vi "Main_02a.vi"() -> ()   [LabVIEW 2020]
uses:
  ENUM RPS Select.ctl
panel:
  in  "Example":string="A Y\nC Y\nC X\nA Y\nC X\nC Y\nB Z\nA Y\nA Y\nC Z\nA Y\nA Y\nA Y\nC Y\nA Y\nA Y\nA Y\nA X\nB X\nA X\nA Y\nC Y\nC X\nA Y\nA Y\nC Y\nA X\nA Y\nB Z\nA Y\nC X\nA Y\nA Y\nC Z\nC Y\nC X\nA Y\nA Z\nA Y\nA Y\nA Y\nA Y\nC Y\nC Y\nB Z\nB Z\nC Y\nB X\nA Y\nA Y\nA Y\nC Z\nA Y\nC X\nA Z\nC Y\nA Y\nA Y\nA Y\nA Y\nA Y\nC X\nA Y\nC Y\nA Y\nC Y\nA Y\nA X\nC Y\nA X\nA Y\nC Y\nC Y\nA Y\nC X\nA Y\nA Y\nA Y\nC X\nA Y\nA Y\nA Y\nC X\nA Y\nC X\nA Y\nA Y\nC Z\nA Y\nA Y\nA Y\nC X\nA Y\nA X\nC Y\nA X\nB Z\nC Y\nA Y\nA Y\nB Z\nC Y\nA Y\nA Z\nC Z\nC Y\nB Z\nA Y\nA Y\nC Y\nA Y\nC X\nA Y\nA Y\nC X\nC X\nC Y\nA Y\nA Y\nC X\nA Y\nA Y\nA Y\nA Y\nC X\nC Y\nA Y\nA Y\nA Y\nC Z\nA Y\nC Y\nA Y\nC X\nC Z\nA Y\nB X\nA Y\nC X\nA Y\nB X\nA Y\nC Z\nA Y\nA Y\nA Y\nA X\nA Y\nA Y\nA Y\nC Y\nA Y\nA Y\nA Y\nA Y\nC Y\nC X\nA Y\nA Y\nA Y\nA Y\nC Y\nA Y\nA Y\nA Y\nC Y\nB X\nA Y\nA Y\nA Y\nA Y\nA Y\nA X\nC Y\nA Y\nC X\nA X\nB Y\nA Y\nC X\nA Y\nC Y\nC Y\nA Z\nC Z\nC X\nB X\nC Y\nA Y\nC Z\nA Z\nA Y\nC X\nA Y\nA Y\nC X\nA Y\nB X\nC X\nA Z\nC Y\nA Y\nC X\nA Y\nA Y\nA Y\nB Z\nC Z\nA Y\nA X\nC X\nA Y\nA Y\nC Y\nA Y\nA Y\nA X\nA X\nC Y\nC X\nB X\nA Y\nA Y\nA Y\nA Y\nB Y\nA Y\nC Y\nA Y\nA X\nB Z\nA X\nC Z\nC X\nC X\nC Y\nC X\nC X\nA X\nC X\nA Y\nC Y\nA X\nC X\nB Z\nC Z\nA Y\nC X\nB Y\nA Z\nC Y\nC X\nA Y\nA Y\nA Y\nC X\nA Y\nA Y\nA Y\nA X\nB Y\nC Y\nC X\nB Z\nA Y\nA Y\nB Y\nA Y\nA Y\nA Y\nC X\nA Y\nA Y\nA Y\nA Y\nA Y\nA Y\nA Y\nA Y\nA Y\nC Y\nC Y\nC Z\nA Y\nC Y\nA Y\nA Y\nA X\nA X\nA Y\nA Y\nC Y\nA Y\nA X\nA Y\nA Y\nC X\nA Y\nC X\nC X\nC Y\nB Y\nA Y\nC X\nA Y\nA Y\nA X\nA Y\nA Y\nA X\nA Y\nB Z\nC Y\nA Y\nA Y\nA Y\nC Y\nC Z\nA Y\nA Y\nA Y\nA Y\nA Y\nC Y\nC Y\nC Y\nC Y\nC Y\nA X\nC Y\nA Y\nA Y\nA Y\nA Y\nC X\nA Y\nC Z\nA Y\nB Y\nA X\nA Y\nA Y\nA Y\nC Y\nC Y\nA X\nC Y\nA Y\nA Y\nA Y\nB Z\nA X\nA Y\nA Y\nA Z\nC Y\nA Y\nC X\nC Y\nC Y\nC Z\nB Y\nC X\nC X\nA Z\nC Y\nA Y\nA Z\nA X\nA Z\nC Y\nC X\nB Z\nA X\nC Y\nA Y\nC Y\nB Z\nA Y\nA Y\nC X\nC X\nC X\nA Y\nB X\nC X\nC Y\nC X\nA X\nA X\nB X\nA Y\nA Y\nA Y\nC X\nA Y\nC Y\nC X\nA Y\nB Z\nA Y\nA Y\nA Y\nB X\nA Y\nA Y\nA Y\nC Y\nA Y\nC X\nC Y\nC Y\nA Y\nB Z\nC Y\nC X\nC Y\nC X\nC X\nC Y\nA Y\nA Z\nA Y\nA Y\nA Y\nA Y\nC Z\nA Y\nA Y\nC Y\nA Y\nA X\nC Z\nC Y\nC X\nC X\nA Y\nA Z\nA Z\nB Y\nA X\nC X\nC X\nA Y\nA Y\nA Y\nC Z\nC X\nC X\nC X\nA Y\nC Z\nA Z\nC X\nC Y\nA X\nC X\nC X\nA Y\nC Y\nC Y\nB X\nB Z\nA Y\nA Y\nA Y\nB Z\nC Y\nA Y\nB Z\nA X\nC Y\nC Y\nB X\nC X\nB Y\nA Y\nB X\nC Z\nA Y\nA Z\nC Z\nC Z\nA Y\nA X\nA Y\nA X\nC Y\nA Y\nA Y\nA Y\nC X\nC X\nC X\nA Y\nA Y\nA Y\nA Y\nA Y\nC Y\nA Y\nC Y\nA Z\nC X\nC Y\nA Y\nA Y\nB Y\nC Y\nA Y\nC Z\nC Z\nA Y\nB Y\nA Y\nA Y\nA X\nC Y\nA Y\nA Y\nA Y\nC Z\nC Y\nC X\nA Y\nA Y\nB Z\nC Y\nC X\nC Z\nA Y\nC Y\nA Y\nA Y\nC X\nC Y\nC Y\nA Y\nC Y\nC X\nC Y\nA Y\nA Y\nA Y\nA Z\nB Z\nA Y\nA Y\nA X\nC Z\nC X\nA Y\nA Y\nA Y\nC X\nC Y\nB Z\nC X\nA Y\nA Y\nA Y\nC Y\nA Y\nC X\nC Z\nC X\nA Y\nA X\nA Y\nC Z\nC X\nB Y\nA Y\nA X\nA Y\nB Y\nA Y\nA Y\nC Y\nC Z\nC Y\nC Y\nC X\nA Y\nA Y\nA X\nA Y\nA Y\nA Z\nA X\nC Y\nA Y\nC Y\nC Y\nC Z\nC Y\nC Y\nA Z\nA Y\nC Z\nC Y\nC Y\nC Y\nB X\nC Y\nA Y\nC X\nA Y\nB X\nC Z\nC Z\nC Y\nA Y\nC X\nA Y\nA Y\nA Y\nA Y\nC Z\nA Z\nA X\nC Y\nC X\nA Y\nA Y\nC X\nC Y\nC Z\nC X\nC Y\nA X\nA Y\nA Y\nB X\nA Y\nA X\nC X\nA Y\nA Y\nA Y\nB Z\nA Z\nB Z\nC X\nB Z\nA Y\nC X\nA Y\nC X\nA Y\nA Y\nC Y\nA Y\nA Y\nB X\nA Y\nC Y\nA Y\nA Y\nA Y\nC Y\nA Y\nA Y\nA Y\nB Y\nA Y\nC Y\nA Y\nA Y\nA Y\nA Y\nC Y\nA X\nB X\nA Y\nB Z\nC X\nA X\nB X\nC Y\nA Y\nB X\nC Y\nA Y\nB X\nA Y\nC X\nB X\nA Y\nA Y\nA Y\nA Y\nC X\nC X\nA Y\nB X\nC Y\nA Y\nA Y\nA Y\nA Y\nB X\nA Y\nB Z\nC X\nA Y\nB Z\nC X\nC Z\nC Z\nB X\nC Y\nA Y\nA Y\nA Y\nA Y\nA Y\nA Y\nC Y\nA Y\nA Y\nA X\nA X\nC X\nA Y\nC Z\nC Y\nA Y\nC X\nA Z\nA Z\nA Y\nC Z\nA Y\nA Y\nA Y\nC Y\nA X\nC X\nC Z\nA Y\nA Y\nC X\nB X\nA Y\nA Z\nC Y\nA Z\nA Y\nA Y\nA Y\nA Y\nA Y\nB X\nA Y\nC Y\nC X\nA Y\nA Y\nC Z\nC Z\nC Y\nA Y\nB Z\nA Y\nA Y\nA Y\nA Y\nA Y\nC X\nA Z\nA Y\nC Y\nA Z\nC X\nA Y\nC X\nA Y\nA Y\nC Z\nC Y\nA Y\nA Z\nC X\nC X\nA Y\nB Z\nA Y\nB X\nC Y\nC X\nC Z\nA Y\nA X\nC X\nC Z\nC Y\nC X\nA Y\nA Y\nA Y\nA Y\nA Y\nA Y\nC Y\nA Y\nC Y\nA Y\nC Y\nB Y\nA Y\nA Y\nA Y\nA Y\nB Z\nC Y\nA Y\nC Y\nA X\nC Y\nA Y\nB Y\nC Y\nC X\nC X\nA Y\nA Y\nA Y\nC X\nA X\nA Y\nA X\nC Y\nA Y\nA Y\nC Y\nC Y\nA Z\nA Y\nA Y\nB X\nA Z\nB X\nA Y\nC Y\nA X\nC Y\nC Z\nB Z\nA Y\nA Y\nC Y\nA Y\nC Z\nA Y\nA X\nA Y\nC Y\nA Y\nA Y\nA Y\nA Y\nA Y\nA Y\nA Y\nA Y\nC X\nC Y\nA Y\nA Z\nA Y\nC X\nA Y\nC Z\nA Y\nC X\nA X\nA Y\nC Y\nA Y\nC X\nA X\nA Y\nA Y\nA Y\nC Y\nA Y\nC Y\nA Y\nB Y\nC Y\nC Y\nA Y\nA Y\nA Y\nA Y\nC Z\nA Y\nC Z\nA Y\nC Y\nB X\nA X\nC Y\nC Z\nA X\nA Z\nA Y\nA X\nC Z\nC Y\nA Z\nC Y\nA X\nA Y\nA Y\nA X\nC Z\nA X\nA Z\nC Y\nA Y\nC Y\nA Z\nB Z\nA Y\nC X\nC X\nA Y\nA Y\nA X\nA Y\nA Y\nA Y\nC X\nA Y\nB X\nA Y\nC X\nA Y\nC Y\nA Y\nC Y\nC Z\nC Y\nC Z\nA Z\nA Y\nC Y\nC Z\nC Z\nA Y\nA Y\nC Y\nA X\nA Y\nC Y\nA Y\nA Y\nA Y\nA X\nA Y\nB Z\nC Y\nC X\nA Y\nC X\nB X\nC Y\nC Y\nA Y\nC Y\nC Y\nA X\nA Y\nA X\nA Y\nA Z\nC Z\nB X\nA Y\nC X\nA Y\nC Z\nA Y\nC Y\nA Z\nA Y\nA Y\nA Y\nC Y\nC Y\nA Y\nA Y\nC Y\nA Y\nC Y\nC Y\nA X\nA Y\nC X\nC Z\nA Y\nA Y\nA Y\nC X\nC X\nC Y\nC Y\nC Z\nA X\nA Y\nC Y\nC Z\nA Y\nB Y\nA Y\nC Z\nC Z\nA Y\nA Y\nA Y\nB Z\nA Y\nA Z\nA X\nC X\nC X\nC Z\nA Y\nC Z\nA Z\nC Y\nC Z\nC X\nC Y\nC X\nA Y\nC Y\nA Z\nA Y\nA Y\nA Y\nA Y\nC Y\nA X\nC X\nA Y\nA Y\nC Z\nB Z\nA Y\nA Y\nC X\nA Y\nC Y\nC Y\nB Z\nA Y\nC Y\nA Y\nC X\nC X\nA Y\nC Y\nA X\nC X\nA Y\nC Z\nA Y\nC X\nA Y\nC X\nA Y\nC Y\nA Y\nC Z\nA Y\nC Z\nA Y\nA Y\nA Y\nC Y\nA Y\nA X\nA Z\nA Y\nC Y\nC Y\nA Y\nA Y\nB Z\nA X\nA X\nC X\nC X\nC Z\nC Z\nA Y\nA Y\nA Y\nA X\nA X\nA Y\nA Z\nC Y\nC Y\nC X\nA Y\nC X\nB X\nA X\nA Z\nA Y\nB X\nA Y\nB Z\nB Z\nA Y\nB X\nC Y\nA Y\nA Y\nC Y\nC Y\nA Y\nA Y\nA Z\nA Y\nC Z\nB X\nA Y\nC Y\nC Y\nA Y\nB X\nC X\nC Y\nA X\nC X\nA Y\nA X\nA Y\nA Y\nB Z\nA X\nC Y\nA Y\nA Z\nB Y\nA Y\nB X\nA Z\nC Y\nC Z\nC Z\nC Z\nC Y\nA Y\nC Y\nC Y\nB Y\nA Y\nC Z\nB Y\nA Y\nA Y\nA Y\nA X\nB Z\nA Y\nC Z\nA Y\nA X\nC Z\nC X\nA Y\nA Y\nA Y\nB Z\nB Z\nA Y\nC Z\nA Y\nA Y\nA Y\nC Y\nC Z\nC X\nA Y\nB Z\nC Y\nB Z\nC X\nC X\nA Y\nA X\nA X\nB Z\nC Y\nC Y\nC X\nA Y\nC X\nC X\nA Y\nC X\nC Z\nA X\nC Y\nC Y\nC Y\nA Y\nA X\nC Y\nA Y\nA Y\nC Y\nC X\nC Y\nB X\nC X\nA Z\nA X\nA Y\nC Y\nA Y\nA X\nC Y\nA Y\nA X\nC X\nA X\nC X\nC Y\nC Y\nA Y\nC X\nA Y\nA X\nC Y\nA Y\nC Z\nA Z\nA Y\nA Y\nA Y\nA Z\nA Y\nB X\nB Z\nC X\nA Z\nC X\nA Y\nA Z\nA X\nC Y\nC Y\nB Z\nA Z\nA Y\nA Y\nA Y\nB X\nC Y\nA Y\nA X\nA Y\nB Z\nB Z\nA Y\nA Y\nA Y\nC X\nC X\nC X\nC Y\nA Y\nC Y\nC Y\nA Y\nA Y\nA Y\nA Y\nC Y\nA Y\nC X\nA Y\nC X\nC Y\nC Y\nC Z\nB X\nA Y\nC Y\nA Y\nC Y\nA Y\nA Y\nA Y\nA Y\nB Z\nC Z\nC Y\nA X\nC Y\nA Y\nC Y\nC Y\nA Y\nB Z\nC Y\nB X\nB X\nA Y\nA Y\nC Y\nC Y\nB X\nA X\nC Y\nC X\nC Y\nA Y\nA Y\nC X\nA X\nA Z\nA Y\nA Z\nA Y\nB X\nA X\nC X\nA X\nC X\nC Z\nA Y\nC X\nC Y\nC X\nC Y\nA Y\nC Y\nA Y\nA Y\nC Y\nC Z\nC X\nA Y\nA Y\nA X\nC Y\nB Z\nA Y\nC Y\nB Z\nC Y\nA Y\nC Y\nA X\nA X\nA Y\nB X\nA Y\nC X\nC Y\nA Y\nA Y\nA Y\nC X\nC Z\nA Y\nC Y\nA Z\nC Y\nA Y\nC Y\nA Y\nC Z\nC Y\nC X\nA Y\nC X\nA Z\nB Z\nA Y\nA X\nA Y\nA Y\nA X\nA Y\nA Y\nA Y\nA Y\nC Y\nC X\nA Y\nA Y\nA Y\nA Y\nA Y\nC Y\nC Y\nC Y\nA X\nA Z\nA Y\nC X\nA Y\nA Y\nC Y\nB Y\nC Y\nA X\nA Y\nA Y\nA Y\nC X\nA X\nC Y\nC Z\nA Y\nB Z\nA Z\nC Y\nA Y\nA Y\nB Z\nA X\nA Y\nC Y\nA Y\nA X\nB X\nC Z\nB X\nA Y\nA Y\nC Y\nA Y\nA Z\nA Y\nA Y\nA Y\nC X\nA Y\nA Z\nA Z\nA Y\nC X\nA Y\nC Z\nC Y\nB X\nC Y\nA Y\nC Z\nB Z\nA Y\nC Y\nA Z\nA Y\nC X\nC Y\nA X\nA Y\nC Z\nA Y\nA Y\nA Y\nA Y\nB Z\nA Z\nC Z\nA X\nA Y\nA Y\nA Y\nA Y\nA Y\nC Y\nC Y\nA Y\nC X\nA Y\nA Y\nA X\nA X\nA Y\nC Y\nC Z\nA Z\nA Y\nA X\nB X\nB X\nB Z\nC X\nC Y\nA Y\nA Y\nA Y\nC Z\nA Y\nA Y\nA Y\nC Y\nC Y\nB Y\nC Z\nB Z\nC Y\nB Z\nA Y\nA X\nC X\nA X\nC X\nB Y\nA Y\nA Z\nA Y\nA X\nA Y\nA Y\nC X\nA Y\nA Y\nC X\nC X\nA Y\nC X\nC Z\nC X\nB Z\nB Z\nB Z\nC Y\nB Z\nC Y\nC Z\nB Y\nA Y\nC Z\nA Y\nC X\nC X\nB Z\nB Y\nA Y\nA Z\nC Y\nC X\nC Y\nA Z\nC X\nC X\nC X\nA Y\nA Y\nC Y\nA Y\nC Y\nC Y\nA Y\nC Y\nC Z\nA Y\nB Y\nC Y\nC X\nA Y\nA Y\nA X\nA Y\nC Y\nB Z\nA Y\nA Y\nA Y\nA Y\nC X\nB X\nA Y\nA Y\nA Y\nA Y\nB X\nA Y\nA Y\nA X\nC Y\nA Y\nA Y\nC X\nA Y\nA Y\nA Y\nC X\nB Y\nA Z\nC Y\nC X\nA Y\nA Z\nB X\nA Y\nA Y\nA X\nC Y\nC Y\nC Y\nA Y\nC Z\nA Y\nA Y\nC Y\nB Z\nA Y\nA Y\nC X\nA X\nA Y\nA Y\nA Y\nB Z\nC Y\nA Y\nC Y\nC Y\nA Y\nA Y\nC Y\nC Y\nA Y\nC Y\nA Y\nB X\nC Y\nA X\nA Z\nA Y\nA Y\nC Y\nC Y\nA Y\nC Z\nA Z\nA Y\nA Y\nC Y\nC Y\nC X\nC Y\nA Y\nC X\nC Y\nA Y\nC X\nC Y\nC Y\nA Y\nA Y\nA Y\nC X\nC Y\nA Y\nA Y\nC Y\nA Y\nC Y\nA Y\nA Y\nC Y\nC Y\nC Y\nA Z\nA Y\nC Y\nC Y\nA Y\nA X\nC X\nA Y\nC Y\nB X\nC Y\nA Y\nA Y\nC Y\nC Y\nA Y\nA Y\nA Y\nB Z\nA Y\nC Y\nA Y\nA Y\nC X\nC Y\nA Y\nA Y\nC Y\nC Y\nC Y\nC Z\nA Y\nA Y\nC X\nA Y\nC Z\nA X\nC X\nB X\nA Y\nC Y\nA Y\nA Y\nA X\nA Y\nA Z\nB Y\nA X\nA Y\nC Y\nC Y\nC X\nA Y\nC Y\nA Y\nC Y\nA Y\nC X\nC X\nA Y\nC Y\nC Z\nC X\nB X\nA Y\nB X\nA Y\nA Y\nC Y\nA Y\nC Y\nA Y\nA Y\nA Y\nA Y\nA X\nA Z\nA Y\nB X\nA Y\nA Y\nC X\nA Y\nC Z\nA Y\nA Y\nC Y\nC X\nC X\nA Y\nA Y\nB X\nC X\nA Y\nC Y\nA Y\nC Y\nA Y\nB Z\nA Y\nC Y\nA Y\nA Y\nA Y\nC Z\nA Y\nA X\nC X\nA X\nA Y\nA Y\nA Y\nC X\nC Y\nC Y\nC Y\nA Y\nA Y\nA Z\nC X\nA Y\nA Y\nA Y\nC Y\nC Y\nA X\nA Y\nC Y\nB Y\nA Y\nA Z\nC X\nA Y\nA Z\nA X\nA Y\nA Y\nA Y\nC Y\nA Y\nA Y\nA X\nC Y\nA X\nB X\nC X\nC Y\nA Y\nA Y\nA Y\nC Y\nA Y\nA Y\nA Y\nA X\nC X\nA Y\nA Y\nA Y\nC Y\nA Y\nB Y\nC Y\nC Y\nC Y\nC Y\nA Y\nA Y\nC Y\nC Y\nA Y\nC Y\nC Y\nA Y\nC Y\nC X\nC X\nC Y\nA X\nC X\nC X\nA Z\nC Y\nC Z\nA Y\nB Z\nA Y\nA Y\nB X\nC Y\nA Y\nC Z\nA Y\nC Z\nA Y\nA Y\nA X\nC Y\nC X\nC X\nC Y\nC X\nA Y\nA Y\nC X\nA Y\nA Z\nB X\nC X\nC Y\nB X\nB Z\nA Y\nA Y\nA Y\nC Y\nA X\nC Y\nC Y\nC X\nA Y\nC X\nA Y\nA X\nC X\nA Y\nA Y\nA X\nC Y\nB Y\nA Y\nA X\nA Y\nC Y\nA X\nC Y\nA Z\nA Y\nA Y\nC Z\nA Z\nC Y\nA Y\nC Y\nA Y\nA Z\nC Y\nC Y\nB Z\nB Y\nC X\nC X\nB Z\nA Y\nA Y\nA Y\nA Y\nA Y\nA Y\nC X\nA Y\nC Y\nA Y\nB Y\nA Y\nA Y\nB X\nA X\nC X\nC Y\nA Y\nC Y\nA Y\nA Y\nA Y\nA Y\nC X\nB Z\nA Z\nC Y\nB Y\nC X\nA Y\nA X\nA Y\nA Y\nC Y\nC Y\nA Y\nA Y\nC Y\nB Z\nC Y\nA X\nC Y\nA Z\nA Y\nA Y\nA Y\nB X\nA Y\nC Y\nC X\nB Y\nC Y\nA Y\nB Y\nA Y\nA Y\nC X\nC Y\nC Y\nA Y\nA Y\nC X\nC X\nC Y\nA Y\nC X\nC X\nB X\nC Y\nA Y\nC Y\nB Z\nA Y\nB X\nC Y\nC X\nA X\nA Y\nC Y\nA Y\nA Y\nA Y\nC X\nA Y\nC X\nC X\nA Y\nC Y\nA Y\nB Z\nC X\nC Y\nC Y\nB X\nA Y\nC Y\nA X\nA X\nB Z\nC X\nA Y\nC Y\nA Y\nA X\nC Y\nA Y\nA Y\nA X\nA X\nA Z\nC Z\nB Y\nC Y\nC X\nA Y\nA Y\nC Y\nA Y\nC Z\nC X\nC X\nC Z\nC Y\nC X\nC X\nA Y\nC Z\nB X\nC Z\nA Y\nA Y\nC Y\nC X\nC Z\nC X\nC X\nC Y\nC X\nC Y\nA Y\nA X\nA Y\nC X\nA Y\nA Y\nA Y\nA Y\nA Z\nC X\nA X\nB X\nA Y\nA Y\nC Z\nC Y\nA Y\nA Y\nC Y\nC Y\nC Y\nA Y\nA Y\nA Y\nB X\nA Y\nB Z\nA Z\nA X\nA X\nC Y\nA Y\nC Z\nA Y\nA Y\nC Y\nA Y\nA X\nC Y\nC Y\nA X\nA Y\nC Y\nA Y\nC X\nA Y\nC X\nA X\nA Y\nA Y\nA Y\nB X\nC Z\nA Z\nB Y\nA Y\nB Z\nB Z\nA Y\nC Z\nB Z\nA Y\nA Y\nA Y\nC Y\nB X\nA Y\nC X\nA Y\nC Z\nC X\nB Y\nC X\nC X\nB X\nC Y\nB Z\nA X\nA Y\nB Y\nC Z\nA Y\nA Z\nA Y\nC X\nA Y\nA Y\nC Y\nC X\nB Y\nB X\nC Y\nB X\nC Y\nA X\nA Z\nA X\nC X\nB Z\nC Y\nC X\nA Y\nA Y\nA X\nB X\nC X\nA Y\nB Y\nC Z\nA Y\nC Y\nA Y\nA Y\nA Y\nB X\nA Y\nC X\nA Y\nA Y\nA Y\nA X\nC X\nA X\nC Z\nC Y\nA Y\nA Y\nC Y\nA X\nC Z\nA Y\nA Y\nA Y\nB Y\nC Y\nC Y\nC Z\nC Z\nC Z\nA Y\nC Y\nA Y\nA Y\nA Y\nA Y\nA Y\nB Y\nC Y\nC Y\nA X\nC Z\nC Y\nA Y\nA Y\nA Y\nC X\nA Z\nA Y\nA Y\nA X\nA Z\nC X\nB Y\nA Y\nA Y\nC Y\nB X\nA Y\nA Y\nC Y\nC Y\nC Z\nA X\nC Y\nC X\nC X\nC Z\nA X\nB Z\nC X\nC X\nC Y\nC X\nC Z\nC X\nC X\nB Z\nB Z\nA Y\nB Z\nA Y\nA Y\nA Y\nB X\nC X\nA Y\nC Z\nA Z\nA X\nA Y\nB Y\nB X\nB Z\nA Y\nA X\nA X\nA Y\nC X\nB X\nA Y\nC Y\nA Y\nA Y\nC X\nC Y\nC X\nC Z\nB X\nC X\nC Z\nA Z\nA X\nA Y\nA Y\nA Y\nC Z\nA Y\nC Y\nC X\nA Y\nA Y\nC X\nC X\nA Y\nC Y\nC Z\nC Y\nC X\nB Y\nC Y\nC X\nA Y\nB X\nC X\nA Y\nA Y\nC Y\nC Z\nA Y\nA Z\nB Y\nA Y\nB X\nC Y\nC Z\nB X\nB X\nC X\nA Y\nB Z\nA Y\nA Y\nA Y\nA Y\nC X\nA Y\nA Y\nC Z\nC X\nB Y\nC Y\nC Y\nA Y\nC X\nB Z\nA Z\nC Y\nA Y\nB Y\nB X\nB Y\nA Z\nC Y\nC Z\nA Y\nC Z\nC X\nA Y\nA Z\nC Z\nA Y\nA Y\nA Y\nC X\nA Y\nC Y\nB Z\nA Y\nC X\nA X\nA Y\nC Y\nC Z\nC Y\nA Y\nC Z\nA Z\nA Y\nC Y\nA Y\nC X\nA Y\nA Y\nB Z\nA Y\nA Y\nA Y\nC Y\nC Y\nC Y\nC X\nC Y\nC X\nB Z\nA Y\nA Y\nA Z\nA Z\nA Y\nA Z\nA Y\nA Y\nA X\nC Z\nA Y\nA Y\nA Y\nC X\nC Y\nC X\nA Y\nA Y\nA Y\nC Y\nC X\nB Y\nA Y\nC Y\nC Y\nA Z\nC Z\nA Y\nA X\nA Y\nA Y\nB X\nA Y\nC Y\nA X\nC Y\nA Y\nA Y\nA X\nC Y\nA X\nB X\nC Y\nA Y\nA Y\nA Y\nA Y\nC Z\nC Y\nC X\nA X\nA Y\nC X\nC Y\nA X\nA X\nB Y\nB Z\nA Y\nC Z\nA X\nC Y\nA X\nA Y\nC Y\nC X\nC Y\nC X\nA Y\nA X\nA Y\nA X\nC Z\nA X\nA Y\nC Y\nC X\nC Y\nC X\nA Y\nC Y\nC X\nA Y\nA Y\nC Y\nC Y\nA Y\nA Z\nC Y\nA Z\nA Y\nC Y\nA Y\nA Y\nC Y\nA Y\nB X\nC X\nC Y\nC X\nA Y\nB Y\nC Z\nA Y\nC X\nA Y"
  out "Score":u32
  in  "Puzzle":string="A Y\nC Y\nC X\nA Y\nC X\nC Y\nB Z\nA Y\nA Y\nC Z\nA Y\nA Y\nA Y\nC Y\nA Y\nA Y\nA Y\nA X\nB X\nA X\nA Y\nC Y\nC X\nA Y\nA Y\nC Y\nA X\nA Y\nB Z\nA Y\nC X\nA Y\nA Y\nC Z\nC Y\nC X\nA Y\nA Z\nA Y\nA Y\nA Y\nA Y\nC Y\nC Y\nB Z\nB Z\nC Y\nB X\nA Y\nA Y\nA Y\nC Z\nA Y\nC X\nA Z\nC Y\nA Y\nA Y\nA Y\nA Y\nA Y\nC X\nA Y\nC Y\nA Y\nC Y\nA Y\nA X\nC Y\nA X\nA Y\nC Y\nC Y\nA Y\nC X\nA Y\nA Y\nA Y\nC X\nA Y\nA Y\nA Y\nC X\nA Y\nC X\nA Y\nA Y\nC Z\nA Y\nA Y\nA Y\nC X\nA Y\nA X\nC Y\nA X\nB Z\nC Y\nA Y\nA Y\nB Z\nC Y\nA Y\nA Z\nC Z\nC Y\nB Z\nA Y\nA Y\nC Y\nA Y\nC X\nA Y\nA Y\nC X\nC X\nC Y\nA Y\nA Y\nC X\nA Y\nA Y\nA Y\nA Y\nC X\nC Y\nA Y\nA Y\nA Y\nC Z\nA Y\nC Y\nA Y\nC X\nC Z\nA Y\nB X\nA Y\nC X\nA Y\nB X\nA Y\nC Z\nA Y\nA Y\nA Y\nA X\nA Y\nA Y\nA Y\nC Y\nA Y\nA Y\nA Y\nA Y\nC Y\nC X\nA Y\nA Y\nA Y\nA Y\nC Y\nA Y\nA Y\nA Y\nC Y\nB X\nA Y\nA Y\nA Y\nA Y\nA Y\nA X\nC Y\nA Y\nC X\nA X\nB Y\nA Y\nC X\nA Y\nC Y\nC Y\nA Z\nC Z\nC X\nB X\nC Y\nA Y\nC Z\nA Z\nA Y\nC X\nA Y\nA Y\nC X\nA Y\nB X\nC X\nA Z\nC Y\nA Y\nC X\nA Y\nA Y\nA Y\nB Z\nC Z\nA Y\nA X\nC X\nA Y\nA Y\nC Y\nA Y\nA Y\nA X\nA X\nC Y\nC X\nB X\nA Y\nA Y\nA Y\nA Y\nB Y\nA Y\nC Y\nA Y\nA X\nB Z\nA X\nC Z\nC X\nC X\nC Y\nC X\nC X\nA X\nC X\nA Y\nC Y\nA X\nC X\nB Z\nC Z\nA Y\nC X\nB Y\nA Z\nC Y\nC X\nA Y\nA Y\nA Y\nC X\nA Y\nA Y\nA Y\nA X\nB Y\nC Y\nC X\nB Z\nA Y\nA Y\nB Y\nA Y\nA Y\nA Y\nC X\nA Y\nA Y\nA Y\nA Y\nA Y\nA Y\nA Y\nA Y\nA Y\nC Y\nC Y\nC Z\nA Y\nC Y\nA Y\nA Y\nA X\nA X\nA Y\nA Y\nC Y\nA Y\nA X\nA Y\nA Y\nC X\nA Y\nC X\nC X\nC Y\nB Y\nA Y\nC X\nA Y\nA Y\nA X\nA Y\nA Y\nA X\nA Y\nB Z\nC Y\nA Y\nA Y\nA Y\nC Y\nC Z\nA Y\nA Y\nA Y\nA Y\nA Y\nC Y\nC Y\nC Y\nC Y\nC Y\nA X\nC Y\nA Y\nA Y\nA Y\nA Y\nC X\nA Y\nC Z\nA Y\nB Y\nA X\nA Y\nA Y\nA Y\nC Y\nC Y\nA X\nC Y\nA Y\nA Y\nA Y\nB Z\nA X\nA Y\nA Y\nA Z\nC Y\nA Y\nC X\nC Y\nC Y\nC Z\nB Y\nC X\nC X\nA Z\nC Y\nA Y\nA Z\nA X\nA Z\nC Y\nC X\nB Z\nA X\nC Y\nA Y\nC Y\nB Z\nA Y\nA Y\nC X\nC X\nC X\nA Y\nB X\nC X\nC Y\nC X\nA X\nA X\nB X\nA Y\nA Y\nA Y\nC X\nA Y\nC Y\nC X\nA Y\nB Z\nA Y\nA Y\nA Y\nB X\nA Y\nA Y\nA Y\nC Y\nA Y\nC X\nC Y\nC Y\nA Y\nB Z\nC Y\nC X\nC Y\nC X\nC X\nC Y\nA Y\nA Z\nA Y\nA Y\nA Y\nA Y\nC Z\nA Y\nA Y\nC Y\nA Y\nA X\nC Z\nC Y\nC X\nC X\nA Y\nA Z\nA Z\nB Y\nA X\nC X\nC X\nA Y\nA Y\nA Y\nC Z\nC X\nC X\nC X\nA Y\nC Z\nA Z\nC X\nC Y\nA X\nC X\nC X\nA Y\nC Y\nC Y\nB X\nB Z\nA Y\nA Y\nA Y\nB Z\nC Y\nA Y\nB Z\nA X\nC Y\nC Y\nB X\nC X\nB Y\nA Y\nB X\nC Z\nA Y\nA Z\nC Z\nC Z\nA Y\nA X\nA Y\nA X\nC Y\nA Y\nA Y\nA Y\nC X\nC X\nC X\nA Y\nA Y\nA Y\nA Y\nA Y\nC Y\nA Y\nC Y\nA Z\nC X\nC Y\nA Y\nA Y\nB Y\nC Y\nA Y\nC Z\nC Z\nA Y\nB Y\nA Y\nA Y\nA X\nC Y\nA Y\nA Y\nA Y\nC Z\nC Y\nC X\nA Y\nA Y\nB Z\nC Y\nC X\nC Z\nA Y\nC Y\nA Y\nA Y\nC X\nC Y\nC Y\nA Y\nC Y\nC X\nC Y\nA Y\nA Y\nA Y\nA Z\nB Z\nA Y\nA Y\nA X\nC Z\nC X\nA Y\nA Y\nA Y\nC X\nC Y\nB Z\nC X\nA Y\nA Y\nA Y\nC Y\nA Y\nC X\nC Z\nC X\nA Y\nA X\nA Y\nC Z\nC X\nB Y\nA Y\nA X\nA Y\nB Y\nA Y\nA Y\nC Y\nC Z\nC Y\nC Y\nC X\nA Y\nA Y\nA X\nA Y\nA Y\nA Z\nA X\nC Y\nA Y\nC Y\nC Y\nC Z\nC Y\nC Y\nA Z\nA Y\nC Z\nC Y\nC Y\nC Y\nB X\nC Y\nA Y\nC X\nA Y\nB X\nC Z\nC Z\nC Y\nA Y\nC X\nA Y\nA Y\nA Y\nA Y\nC Z\nA Z\nA X\nC Y\nC X\nA Y\nA Y\nC X\nC Y\nC Z\nC X\nC Y\nA X\nA Y\nA Y\nB X\nA Y\nA X\nC X\nA Y\nA Y\nA Y\nB Z\nA Z\nB Z\nC X\nB Z\nA Y\nC X\nA Y\nC X\nA Y\nA Y\nC Y\nA Y\nA Y\nB X\nA Y\nC Y\nA Y\nA Y\nA Y\nC Y\nA Y\nA Y\nA Y\nB Y\nA Y\nC Y\nA Y\nA Y\nA Y\nA Y\nC Y\nA X\nB X\nA Y\nB Z\nC X\nA X\nB X\nC Y\nA Y\nB X\nC Y\nA Y\nB X\nA Y\nC X\nB X\nA Y\nA Y\nA Y\nA Y\nC X\nC X\nA Y\nB X\nC Y\nA Y\nA Y\nA Y\nA Y\nB X\nA Y\nB Z\nC X\nA Y\nB Z\nC X\nC Z\nC Z\nB X\nC Y\nA Y\nA Y\nA Y\nA Y\nA Y\nA Y\nC Y\nA Y\nA Y\nA X\nA X\nC X\nA Y\nC Z\nC Y\nA Y\nC X\nA Z\nA Z\nA Y\nC Z\nA Y\nA Y\nA Y\nC Y\nA X\nC X\nC Z\nA Y\nA Y\nC X\nB X\nA Y\nA Z\nC Y\nA Z\nA Y\nA Y\nA Y\nA Y\nA Y\nB X\nA Y\nC Y\nC X\nA Y\nA Y\nC Z\nC Z\nC Y\nA Y\nB Z\nA Y\nA Y\nA Y\nA Y\nA Y\nC X\nA Z\nA Y\nC Y\nA Z\nC X\nA Y\nC X\nA Y\nA Y\nC Z\nC Y\nA Y\nA Z\nC X\nC X\nA Y\nB Z\nA Y\nB X\nC Y\nC X\nC Z\nA Y\nA X\nC X\nC Z\nC Y\nC X\nA Y\nA Y\nA Y\nA Y\nA Y\nA Y\nC Y\nA Y\nC Y\nA Y\nC Y\nB Y\nA Y\nA Y\nA Y\nA Y\nB Z\nC Y\nA Y\nC Y\nA X\nC Y\nA Y\nB Y\nC Y\nC X\nC X\nA Y\nA Y\nA Y\nC X\nA X\nA Y\nA X\nC Y\nA Y\nA Y\nC Y\nC Y\nA Z\nA Y\nA Y\nB X\nA Z\nB X\nA Y\nC Y\nA X\nC Y\nC Z\nB Z\nA Y\nA Y\nC Y\nA Y\nC Z\nA Y\nA X\nA Y\nC Y\nA Y\nA Y\nA Y\nA Y\nA Y\nA Y\nA Y\nA Y\nC X\nC Y\nA Y\nA Z\nA Y\nC X\nA Y\nC Z\nA Y\nC X\nA X\nA Y\nC Y\nA Y\nC X\nA X\nA Y\nA Y\nA Y\nC Y\nA Y\nC Y\nA Y\nB Y\nC Y\nC Y\nA Y\nA Y\nA Y\nA Y\nC Z\nA Y\nC Z\nA Y\nC Y\nB X\nA X\nC Y\nC Z\nA X\nA Z\nA Y\nA X\nC Z\nC Y\nA Z\nC Y\nA X\nA Y\nA Y\nA X\nC Z\nA X\nA Z\nC Y\nA Y\nC Y\nA Z\nB Z\nA Y\nC X\nC X\nA Y\nA Y\nA X\nA Y\nA Y\nA Y\nC X\nA Y\nB X\nA Y\nC X\nA Y\nC Y\nA Y\nC Y\nC Z\nC Y\nC Z\nA Z\nA Y\nC Y\nC Z\nC Z\nA Y\nA Y\nC Y\nA X\nA Y\nC Y\nA Y\nA Y\nA Y\nA X\nA Y\nB Z\nC Y\nC X\nA Y\nC X\nB X\nC Y\nC Y\nA Y\nC Y\nC Y\nA X\nA Y\nA X\nA Y\nA Z\nC Z\nB X\nA Y\nC X\nA Y\nC Z\nA Y\nC Y\nA Z\nA Y\nA Y\nA Y\nC Y\nC Y\nA Y\nA Y\nC Y\nA Y\nC Y\nC Y\nA X\nA Y\nC X\nC Z\nA Y\nA Y\nA Y\nC X\nC X\nC Y\nC Y\nC Z\nA X\nA Y\nC Y\nC Z\nA Y\nB Y\nA Y\nC Z\nC Z\nA Y\nA Y\nA Y\nB Z\nA Y\nA Z\nA X\nC X\nC X\nC Z\nA Y\nC Z\nA Z\nC Y\nC Z\nC X\nC Y\nC X\nA Y\nC Y\nA Z\nA Y\nA Y\nA Y\nA Y\nC Y\nA X\nC X\nA Y\nA Y\nC Z\nB Z\nA Y\nA Y\nC X\nA Y\nC Y\nC Y\nB Z\nA Y\nC Y\nA Y\nC X\nC X\nA Y\nC Y\nA X\nC X\nA Y\nC Z\nA Y\nC X\nA Y\nC X\nA Y\nC Y\nA Y\nC Z\nA Y\nC Z\nA Y\nA Y\nA Y\nC Y\nA Y\nA X\nA Z\nA Y\nC Y\nC Y\nA Y\nA Y\nB Z\nA X\nA X\nC X\nC X\nC Z\nC Z\nA Y\nA Y\nA Y\nA X\nA X\nA Y\nA Z\nC Y\nC Y\nC X\nA Y\nC X\nB X\nA X\nA Z\nA Y\nB X\nA Y\nB Z\nB Z\nA Y\nB X\nC Y\nA Y\nA Y\nC Y\nC Y\nA Y\nA Y\nA Z\nA Y\nC Z\nB X\nA Y\nC Y\nC Y\nA Y\nB X\nC X\nC Y\nA X\nC X\nA Y\nA X\nA Y\nA Y\nB Z\nA X\nC Y\nA Y\nA Z\nB Y\nA Y\nB X\nA Z\nC Y\nC Z\nC Z\nC Z\nC Y\nA Y\nC Y\nC Y\nB Y\nA Y\nC Z\nB Y\nA Y\nA Y\nA Y\nA X\nB Z\nA Y\nC Z\nA Y\nA X\nC Z\nC X\nA Y\nA Y\nA Y\nB Z\nB Z\nA Y\nC Z\nA Y\nA Y\nA Y\nC Y\nC Z\nC X\nA Y\nB Z\nC Y\nB Z\nC X\nC X\nA Y\nA X\nA X\nB Z\nC Y\nC Y\nC X\nA Y\nC X\nC X\nA Y\nC X\nC Z\nA X\nC Y\nC Y\nC Y\nA Y\nA X\nC Y\nA Y\nA Y\nC Y\nC X\nC Y\nB X\nC X\nA Z\nA X\nA Y\nC Y\nA Y\nA X\nC Y\nA Y\nA X\nC X\nA X\nC X\nC Y\nC Y\nA Y\nC X\nA Y\nA X\nC Y\nA Y\nC Z\nA Z\nA Y\nA Y\nA Y\nA Z\nA Y\nB X\nB Z\nC X\nA Z\nC X\nA Y\nA Z\nA X\nC Y\nC Y\nB Z\nA Z\nA Y\nA Y\nA Y\nB X\nC Y\nA Y\nA X\nA Y\nB Z\nB Z\nA Y\nA Y\nA Y\nC X\nC X\nC X\nC Y\nA Y\nC Y\nC Y\nA Y\nA Y\nA Y\nA Y\nC Y\nA Y\nC X\nA Y\nC X\nC Y\nC Y\nC Z\nB X\nA Y\nC Y\nA Y\nC Y\nA Y\nA Y\nA Y\nA Y\nB Z\nC Z\nC Y\nA X\nC Y\nA Y\nC Y\nC Y\nA Y\nB Z\nC Y\nB X\nB X\nA Y\nA Y\nC Y\nC Y\nB X\nA X\nC Y\nC X\nC Y\nA Y\nA Y\nC X\nA X\nA Z\nA Y\nA Z\nA Y\nB X\nA X\nC X\nA X\nC X\nC Z\nA Y\nC X\nC Y\nC X\nC Y\nA Y\nC Y\nA Y\nA Y\nC Y\nC Z\nC X\nA Y\nA Y\nA X\nC Y\nB Z\nA Y\nC Y\nB Z\nC Y\nA Y\nC Y\nA X\nA X\nA Y\nB X\nA Y\nC X\nC Y\nA Y\nA Y\nA Y\nC X\nC Z\nA Y\nC Y\nA Z\nC Y\nA Y\nC Y\nA Y\nC Z\nC Y\nC X\nA Y\nC X\nA Z\nB Z\nA Y\nA X\nA Y\nA Y\nA X\nA Y\nA Y\nA Y\nA Y\nC Y\nC X\nA Y\nA Y\nA Y\nA Y\nA Y\nC Y\nC Y\nC Y\nA X\nA Z\nA Y\nC X\nA Y\nA Y\nC Y\nB Y\nC Y\nA X\nA Y\nA Y\nA Y\nC X\nA X\nC Y\nC Z\nA Y\nB Z\nA Z\nC Y\nA Y\nA Y\nB Z\nA X\nA Y\nC Y\nA Y\nA X\nB X\nC Z\nB X\nA Y\nA Y\nC Y\nA Y\nA Z\nA Y\nA Y\nA Y\nC X\nA Y\nA Z\nA Z\nA Y\nC X\nA Y\nC Z\nC Y\nB X\nC Y\nA Y\nC Z\nB Z\nA Y\nC Y\nA Z\nA Y\nC X\nC Y\nA X\nA Y\nC Z\nA Y\nA Y\nA Y\nA Y\nB Z\nA Z\nC Z\nA X\nA Y\nA Y\nA Y\nA Y\nA Y\nC Y\nC Y\nA Y\nC X\nA Y\nA Y\nA X\nA X\nA Y\nC Y\nC Z\nA Z\nA Y\nA X\nB X\nB X\nB Z\nC X\nC Y\nA Y\nA Y\nA Y\nC Z\nA Y\nA Y\nA Y\nC Y\nC Y\nB Y\nC Z\nB Z\nC Y\nB Z\nA Y\nA X\nC X\nA X\nC X\nB Y\nA Y\nA Z\nA Y\nA X\nA Y\nA Y\nC X\nA Y\nA Y\nC X\nC X\nA Y\nC X\nC Z\nC X\nB Z\nB Z\nB Z\nC Y\nB Z\nC Y\nC Z\nB Y\nA Y\nC Z\nA Y\nC X\nC X\nB Z\nB Y\nA Y\nA Z\nC Y\nC X\nC Y\nA Z\nC X\nC X\nC X\nA Y\nA Y\nC Y\nA Y\nC Y\nC Y\nA Y\nC Y\nC Z\nA Y\nB Y\nC Y\nC X\nA Y\nA Y\nA X\nA Y\nC Y\nB Z\nA Y\nA Y\nA Y\nA Y\nC X\nB X\nA Y\nA Y\nA Y\nA Y\nB X\nA Y\nA Y\nA X\nC Y\nA Y\nA Y\nC X\nA Y\nA Y\nA Y\nC X\nB Y\nA Z\nC Y\nC X\nA Y\nA Z\nB X\nA Y\nA Y\nA X\nC Y\nC Y\nC Y\nA Y\nC Z\nA Y\nA Y\nC Y\nB Z\nA Y\nA Y\nC X\nA X\nA Y\nA Y\nA Y\nB Z\nC Y\nA Y\nC Y\nC Y\nA Y\nA Y\nC Y\nC Y\nA Y\nC Y\nA Y\nB X\nC Y\nA X\nA Z\nA Y\nA Y\nC Y\nC Y\nA Y\nC Z\nA Z\nA Y\nA Y\nC Y\nC Y\nC X\nC Y\nA Y\nC X\nC Y\nA Y\nC X\nC Y\nC Y\nA Y\nA Y\nA Y\nC X\nC Y\nA Y\nA Y\nC Y\nA Y\nC Y\nA Y\nA Y\nC Y\nC Y\nC Y\nA Z\nA Y\nC Y\nC Y\nA Y\nA X\nC X\nA Y\nC Y\nB X\nC Y\nA Y\nA Y\nC Y\nC Y\nA Y\nA Y\nA Y\nB Z\nA Y\nC Y\nA Y\nA Y\nC X\nC Y\nA Y\nA Y\nC Y\nC Y\nC Y\nC Z\nA Y\nA Y\nC X\nA Y\nC Z\nA X\nC X\nB X\nA Y\nC Y\nA Y\nA Y\nA X\nA Y\nA Z\nB Y\nA X\nA Y\nC Y\nC Y\nC X\nA Y\nC Y\nA Y\nC Y\nA Y\nC X\nC X\nA Y\nC Y\nC Z\nC X\nB X\nA Y\nB X\nA Y\nA Y\nC Y\nA Y\nC Y\nA Y\nA Y\nA Y\nA Y\nA X\nA Z\nA Y\nB X\nA Y\nA Y\nC X\nA Y\nC Z\nA Y\nA Y\nC Y\nC X\nC X\nA Y\nA Y\nB X\nC X\nA Y\nC Y\nA Y\nC Y\nA Y\nB Z\nA Y\nC Y\nA Y\nA Y\nA Y\nC Z\nA Y\nA X\nC X\nA X\nA Y\nA Y\nA Y\nC X\nC Y\nC Y\nC Y\nA Y\nA Y\nA Z\nC X\nA Y\nA Y\nA Y\nC Y\nC Y\nA X\nA Y\nC Y\nB Y\nA Y\nA Z\nC X\nA Y\nA Z\nA X\nA Y\nA Y\nA Y\nC Y\nA Y\nA Y\nA X\nC Y\nA X\nB X\nC X\nC Y\nA Y\nA Y\nA Y\nC Y\nA Y\nA Y\nA Y\nA X\nC X\nA Y\nA Y\nA Y\nC Y\nA Y\nB Y\nC Y\nC Y\nC Y\nC Y\nA Y\nA Y\nC Y\nC Y\nA Y\nC Y\nC Y\nA Y\nC Y\nC X\nC X\nC Y\nA X\nC X\nC X\nA Z\nC Y\nC Z\nA Y\nB Z\nA Y\nA Y\nB X\nC Y\nA Y\nC Z\nA Y\nC Z\nA Y\nA Y\nA X\nC Y\nC X\nC X\nC Y\nC X\nA Y\nA Y\nC X\nA Y\nA Z\nB X\nC X\nC Y\nB X\nB Z\nA Y\nA Y\nA Y\nC Y\nA X\nC Y\nC Y\nC X\nA Y\nC X\nA Y\nA X\nC X\nA Y\nA Y\nA X\nC Y\nB Y\nA Y\nA X\nA Y\nC Y\nA X\nC Y\nA Z\nA Y\nA Y\nC Z\nA Z\nC Y\nA Y\nC Y\nA Y\nA Z\nC Y\nC Y\nB Z\nB Y\nC X\nC X\nB Z\nA Y\nA Y\nA Y\nA Y\nA Y\nA Y\nC X\nA Y\nC Y\nA Y\nB Y\nA Y\nA Y\nB X\nA X\nC X\nC Y\nA Y\nC Y\nA Y\nA Y\nA Y\nA Y\nC X\nB Z\nA Z\nC Y\nB Y\nC X\nA Y\nA X\nA Y\nA Y\nC Y\nC Y\nA Y\nA Y\nC Y\nB Z\nC Y\nA X\nC Y\nA Z\nA Y\nA Y\nA Y\nB X\nA Y\nC Y\nC X\nB Y\nC Y\nA Y\nB Y\nA Y\nA Y\nC X\nC Y\nC Y\nA Y\nA Y\nC X\nC X\nC Y\nA Y\nC X\nC X\nB X\nC Y\nA Y\nC Y\nB Z\nA Y\nB X\nC Y\nC X\nA X\nA Y\nC Y\nA Y\nA Y\nA Y\nC X\nA Y\nC X\nC X\nA Y\nC Y\nA Y\nB Z\nC X\nC Y\nC Y\nB X\nA Y\nC Y\nA X\nA X\nB Z\nC X\nA Y\nC Y\nA Y\nA X\nC Y\nA Y\nA Y\nA X\nA X\nA Z\nC Z\nB Y\nC Y\nC X\nA Y\nA Y\nC Y\nA Y\nC Z\nC X\nC X\nC Z\nC Y\nC X\nC X\nA Y\nC Z\nB X\nC Z\nA Y\nA Y\nC Y\nC X\nC Z\nC X\nC X\nC Y\nC X\nC Y\nA Y\nA X\nA Y\nC X\nA Y\nA Y\nA Y\nA Y\nA Z\nC X\nA X\nB X\nA Y\nA Y\nC Z\nC Y\nA Y\nA Y\nC Y\nC Y\nC Y\nA Y\nA Y\nA Y\nB X\nA Y\nB Z\nA Z\nA X\nA X\nC Y\nA Y\nC Z\nA Y\nA Y\nC Y\nA Y\nA X\nC Y\nC Y\nA X\nA Y\nC Y\nA Y\nC X\nA Y\nC X\nA X\nA Y\nA Y\nA Y\nB X\nC Z\nA Z\nB Y\nA Y\nB Z\nB Z\nA Y\nC Z\nB Z\nA Y\nA Y\nA Y\nC Y\nB X\nA Y\nC X\nA Y\nC Z\nC X\nB Y\nC X\nC X\nB X\nC Y\nB Z\nA X\nA Y\nB Y\nC Z\nA Y\nA Z\nA Y\nC X\nA Y\nA Y\nC Y\nC X\nB Y\nB X\nC Y\nB X\nC Y\nA X\nA Z\nA X\nC X\nB Z\nC Y\nC X\nA Y\nA Y\nA X\nB X\nC X\nA Y\nB Y\nC Z\nA Y\nC Y\nA Y\nA Y\nA Y\nB X\nA Y\nC X\nA Y\nA Y\nA Y\nA X\nC X\nA X\nC Z\nC Y\nA Y\nA Y\nC Y\nA X\nC Z\nA Y\nA Y\nA Y\nB Y\nC Y\nC Y\nC Z\nC Z\nC Z\nA Y\nC Y\nA Y\nA Y\nA Y\nA Y\nA Y\nB Y\nC Y\nC Y\nA X\nC Z\nC Y\nA Y\nA Y\nA Y\nC X\nA Z\nA Y\nA Y\nA X\nA Z\nC X\nB Y\nA Y\nA Y\nC Y\nB X\nA Y\nA Y\nC Y\nC Y\nC Z\nA X\nC Y\nC X\nC X\nC Z\nA X\nB Z\nC X\nC X\nC Y\nC X\nC Z\nC X\nC X\nB Z\nB Z\nA Y\nB Z\nA Y\nA Y\nA Y\nB X\nC X\nA Y\nC Z\nA Z\nA X\nA Y\nB Y\nB X\nB Z\nA Y\nA X\nA X\nA Y\nC X\nB X\nA Y\nC Y\nA Y\nA Y\nC X\nC Y\nC X\nC Z\nB X\nC X\nC Z\nA Z\nA X\nA Y\nA Y\nA Y\nC Z\nA Y\nC Y\nC X\nA Y\nA Y\nC X\nC X\nA Y\nC Y\nC Z\nC Y\nC X\nB Y\nC Y\nC X\nA Y\nB X\nC X\nA Y\nA Y\nC Y\nC Z\nA Y\nA Z\nB Y\nA Y\nB X\nC Y\nC Z\nB X\nB X\nC X\nA Y\nB Z\nA Y\nA Y\nA Y\nA Y\nC X\nA Y\nA Y\nC Z\nC X\nB Y\nC Y\nC Y\nA Y\nC X\nB Z\nA Z\nC Y\nA Y\nB Y\nB X\nB Y\nA Z\nC Y\nC Z\nA Y\nC Z\nC X\nA Y\nA Z\nC Z\nA Y\nA Y\nA Y\nC X\nA Y\nC Y\nB Z\nA Y\nC X\nA X\nA Y\nC Y\nC Z\nC Y\nA Y\nC Z\nA Z\nA Y\nC Y\nA Y\nC X\nA Y\nA Y\nB Z\nA Y\nA Y\nA Y\nC Y\nC Y\nC Y\nC X\nC Y\nC X\nB Z\nA Y\nA Y\nA Z\nA Z\nA Y\nA Z\nA Y\nA Y\nA X\nC Z\nA Y\nA Y\nA Y\nC X\nC Y\nC X\nA Y\nA Y\nA Y\nC Y\nC X\nB Y\nA Y\nC Y\nC Y\nA Z\nC Z\nA Y\nA X\nA Y\nA Y\nB X\nA Y\nC Y\nA X\nC Y\nA Y\nA Y\nA X\nC Y\nA X\nB X\nC Y\nA Y\nA Y\nA Y\nA Y\nC Z\nC Y\nC X\nA X\nA Y\nC X\nC Y\nA X\nA X\nB Y\nB Z\nA Y\nC Z\nA X\nC Y\nA X\nA Y\nC Y\nC X\nC Y\nC X\nA Y\nA X\nA Y\nA X\nC Z\nA X\nA Y\nC Y\nC X\nC Y\nC X\nA Y\nC Y\nC X\nA Y\nA Y\nC Y\nC Y\nA Y\nA Z\nC Y\nA Z\nA Y\nC Y\nA Y\nA Y\nC Y\nA Y\nB X\nC X\nC Y\nC X\nA Y\nB Y\nC Z\nA Y\nC X\nA Y"
  # "--- Day 2: Rock Paper Scissors ---\nThe Elves begin to set up camp on the beach. To decide whose tent gets to be closest to the snack storage, a giant Rock Paper Scissors tournament is already in progress.\n\nRock Paper Scissors is a game between two players. Each game contains many rounds; in each round, the players each simultaneously choose one of Rock, Paper, or Scissors using a hand shape. Then, a winner for that round is selected: Rock defeats Scissors, Scissors defeats Paper, and Paper defeats Rock. If both players choose the same shape, the round instead ends in a draw.\n\nAppreciative of your help yesterday, one Elf gives you an encrypted strategy guide (your puzzle input) that they say will be sure to help you win. \"The first column is what your opponent is going to play: A for Rock, B for Paper, and C for Scissors. The second column--\" Suddenly, the Elf is called away to help with someone's tent.\n\nThe second column, you reason, must be what you should play in response: X for Rock, Y for Paper, and Z for Scissors. Winning every time would be suspicious, so the responses must have been carefully chosen.\n\nThe winner of the whole tournament is the player with the highest score. Your total score is the sum of your scores for each round. The score for a single round is the score for the shape you selected (1 for Rock, 2 for Paper, and 3 for Scissors) plus the score for the outcome of the round (0 if you lost, 3 if the round was a draw, and 6 if you won).\n\nSince you can't be sure if the Elf is trying to help you or trick you, you should calculate the score you would get if you were to follow the strategy guide.\n\nFor example, suppose you were given the following strategy guide:\n\nA Y\nB X\nC Z\nThis strategy guide predicts and recommends the following:\n\nIn the first round, your opponent will choose Rock (A), and you should choose Paper (Y). This ends in a win for you with a score of 8 (2 because you chose Paper + 6 because you won).\nIn the second round, your opponent will choose Paper (B), and you should choose Rock (X). This ends in a loss for you with a score of 1 (1 + 0).\nThe third round is a draw with both players choosing Scissors, giving you a score of 3 + 3 = 6.\nIn this example, if you were to follow the strategy guide, you would get a total score of 15 (8 + 1 + 6).\n\nWhat would your total score be if everything goes exactly according to your strategy guide?"
  # "14531"
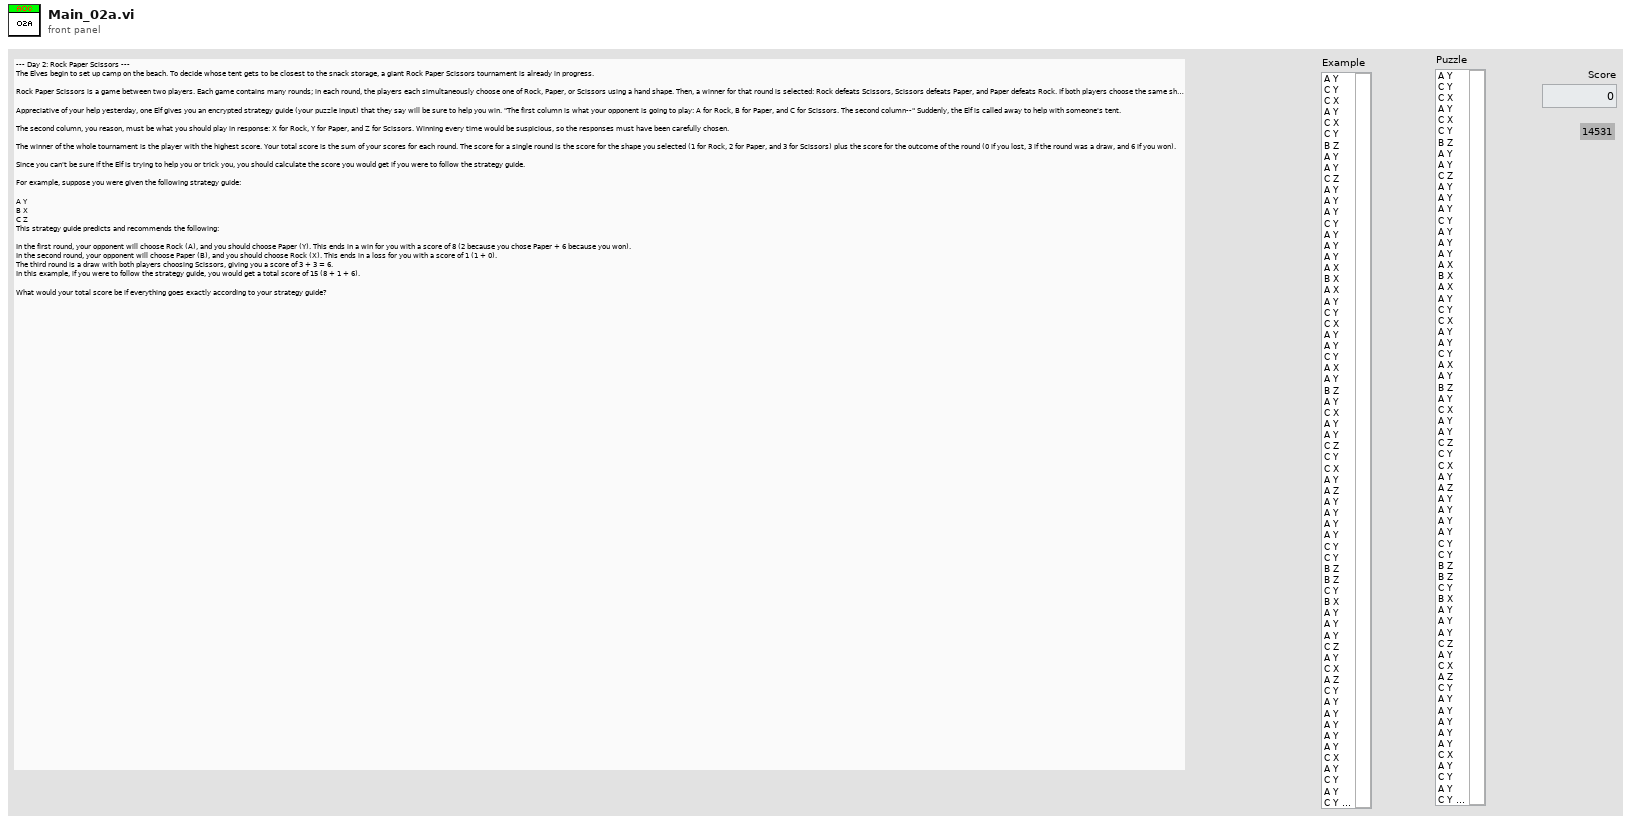
[diagram p1: front panel]
types:
  T1 = typedef "ENUM RPS Select.ctl" = enum16{"A", "B", "C", "X", "Y", "Z"}
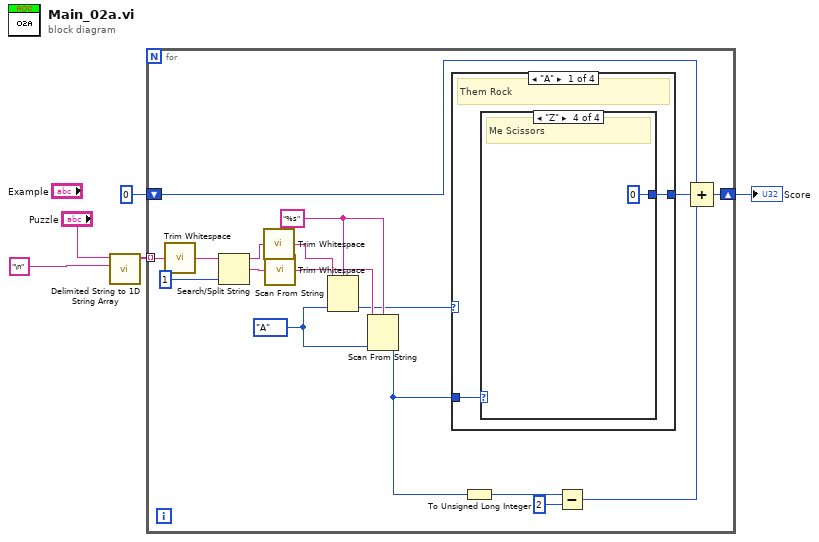
[diagram p0: block diagram]
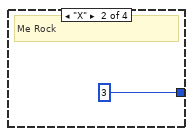
[diagram p3: hidden frame]
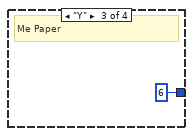
[diagram p4: hidden frame]
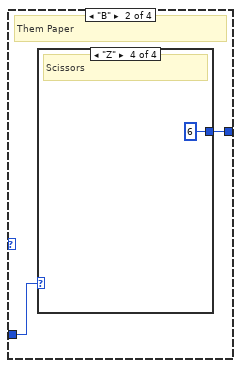
[diagram p5: hidden frame]
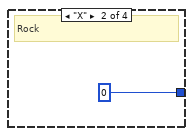
[diagram p7: hidden frame]
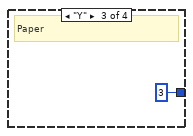
[diagram p8: hidden frame]
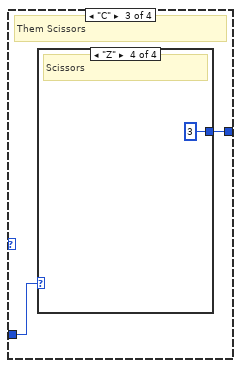
[diagram p9: hidden frame]
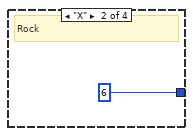
[diagram p11: hidden frame]
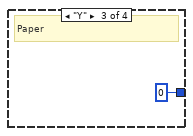
[diagram p12: hidden frame]
diagram:
  n1 = call <vilib>:"Delimited String to 1D String Array.vi"("delimiter"="\n", "delimited string"="Puzzle") -> ("string array"=w4:string[])  [unwired: 9 in]
  n2 = for {
    tunnel: w4 -> [w22] mode=indexing
    shift-right: [w13] -> w3
    shift-left: u32 0 -> [w12]
    w18 = "%s" ("format string")
    w19 = ENUM_RPS_Select."A" ("Select")
    n3 = call <vilib>:"Trim Whitespace.vi"("string"=w22) -> ("trimmed string"=w20:string)  [unwired: 1 in]
    n4 = Search/Split String(string=w20, offset (0)=1) -> (substring before match=w17:string, match + rest of string=w15:string)  [unwired: 1 in, 1 out]
    n5 = call <vilib>:"Trim Whitespace.vi"("string"=w17) -> ("trimmed string"=w16:string)  [unwired: 1 in]
    n6 = call <vilib>:"Trim Whitespace.vi"("string"=w15) -> ("trimmed string"=w14:string)  [unwired: 1 in]
    n7 = Scan From String(format string=w18, input string=w16, default 1=w19) -> (output 1=w9:T1)  [unwired: 2 in, 3 out]
    n8 = Scan From String(format string=w18, input string=w14, default 1=w19) -> (output 1=w6:T1)  [unwired: 2 in, 3 out]
    n9 = case shown="\"A\"" w9 {
      tunnel: w6 -> [w24 w29 w34 _]
      tunnel: [w23 w28 w33 _] -> w7
      frame "A" {
        # "Them Rock"
        n10 = case shown="\"Z\"" w24 {
          tunnel: [_ u32 3 u32 6 u32 0] -> w23
          frame "A".."C" {
          }
          frame "X" {
            # "Me Rock"
          }
          frame "Y" {
            # "Me Paper"
          }
          frame "Z" {
            # "Me Scissors"
          }
        }
      }
      frame "B" {
        # "Them Paper"
        n11 = case shown="\"Z\"" w29 {
          tunnel: [_ u32 0 u32 3 u32 6] -> w28
          frame "A".."C" {
          }
          frame "X" {
            # "Rock"
          }
          frame "Y" {
            # "Paper"
          }
          frame "Z" {
            # "Scissors"
          }
        }
      }
      frame "C" {
        # "Them Scissors"
        n12 = case shown="\"Z\"" w34 {
          tunnel: [_ u32 6 u32 0 u32 3] -> w33
          frame "A".."C" {
          }
          frame "X" {
            # "Rock"
          }
          frame "Y" {
            # "Paper"
          }
          frame "Z" {
            # "Scissors"
          }
        }
      }
      frame "X".."Z" {
      }
    }
    n13 = To Unsigned Long Integer(number=w6) -> (unsigned 32bit integer=w11:u32)
    n14 = Subtract(x=w11, y=u32 2) -> (x-y=w8:u32)
    n15 = Compound Arithmetic op=ADD(w12, w7, w8) -> (w13:u32)
  }
  "Score" <- w3
